vi "RT Read analogue FIFO queue data.vi"(9 "FIFO parameters":T2, 11 "RT Queues":T1) -> ()   [LabVIEW 2018]
doc: "This loop receives data from the FPGA via the FIFO\n\nThis loop performs no processing and just reads data from the FIFO and passes it onto the processing loop.\n\nThis is a mini state-machine with three states:\n* initialise - set parameters and reset variables to initial conditions\n* connect - check for FPGA FIFO connection\n* read data - read data on FIFO and stream to data processing loop\n\nInitial parameters are received when the loop is first called and therefore a RT machine reset is required to use different parameters"
uses:
  Type Defs/Analogue loop data.ctl
  Type Defs/FPGA reference.ctl
  Type Defs/Queues cluster.ctl
  ICL-LabVIEW_General/Message Scheduler/message scheduler.lvclass
  Analogue FIFO loop/Analogue FIFO loop states.ctl
  Queue VIs/De-queue RT FIFO loop element.vi
  Queue VIs/En-queue RT data element.vi
types:
  T1 = typedef "Queues cluster.ctl" = cluster{"RT Message":refnum<queue>, "RT Comms":refnum<queue>, "RT Data":refnum<queue>, "RT FIFO":refnum<queue>, "message scheduler":refnum<class "message scheduler.lvclass">}
  T2 = typedef "Analogue loop data.ctl" = cluster{"Params":cluster{"FPGA ref":T3, "Total Channels":u32}, "Variables":cluster{"FIFO wait counter":u16, "FIFO read trigger":u32}}
  T3 = typedef "FPGA reference.ctl" = refnum<k20>
  T4 = typedef "Analogue FIFO loop states.ctl" = enum16{"init", "message", "read", "stop"}
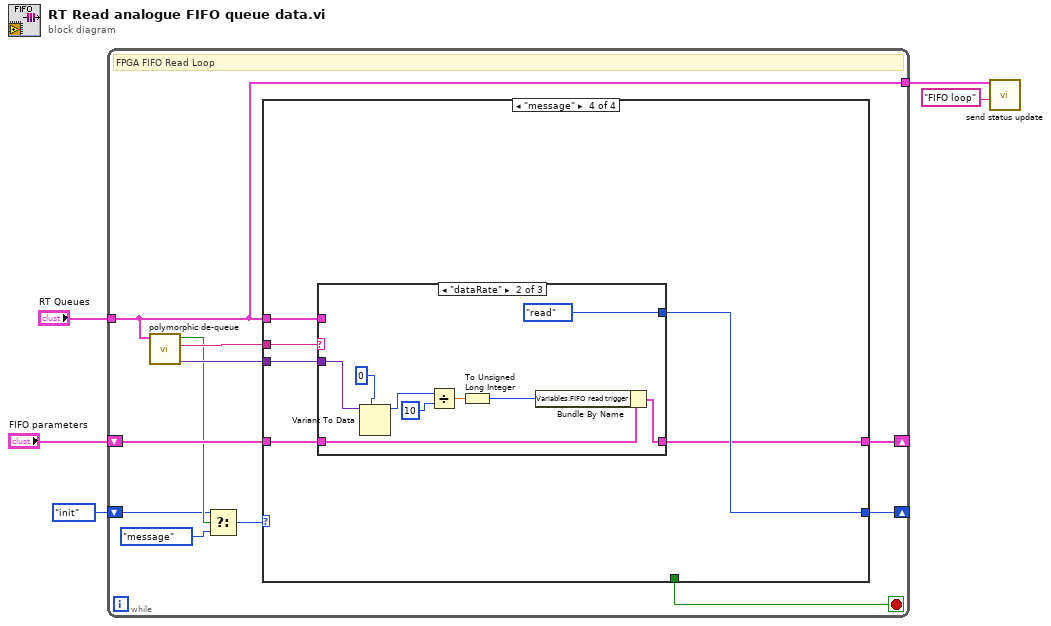
[diagram p0: block diagram]
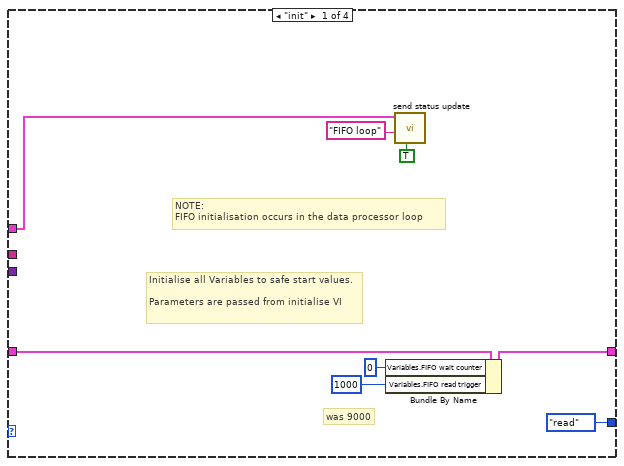
[diagram p2: hidden frame]
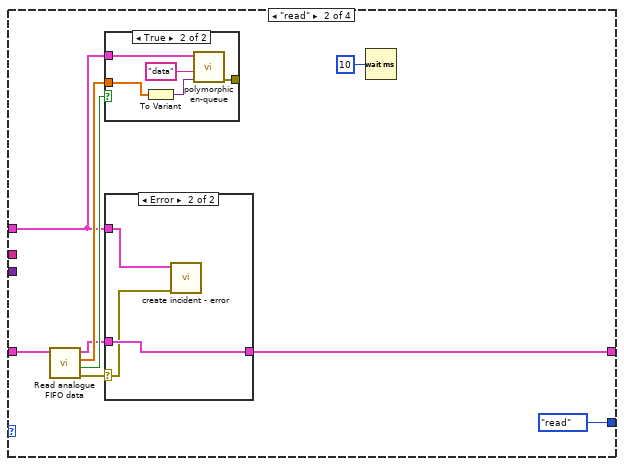
[diagram p3: hidden frame]
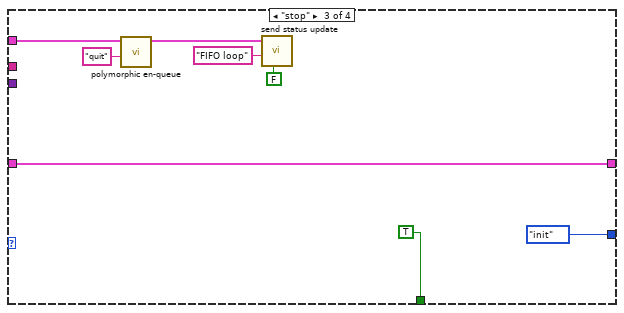
[diagram p6: hidden frame]
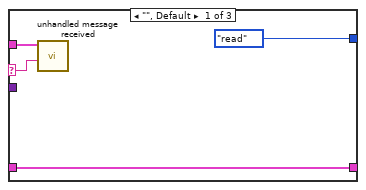
[diagram p7: hidden frame]
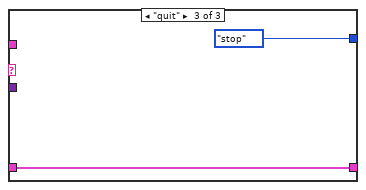
[diagram p8: hidden frame]
diagram:
  n1 = while {
    tunnel: "RT Queues" -> [w9]
    shift-right: [w16] -> _
    shift-left: Analogue_FIFO_loop_states."init" -> [w7]
    shift-right: [w15] -> _
    shift-left: "FIFO parameters" -> [w14]
    tunnel: [w9] -> w1
    stop <- w13 stop-if-true
    # "FPGA FIFO Read Loop"
    n2 = call-poly "polymorphic de-queue.vi"("RT Queues"=w9) -> ("Data"=w11:variant, "Message"=w10:string, "timed out?"=w8:bool)  [unwired: 7 in, 1 out]
    n3 = Select(t=w7, s=w8, f=Analogue_FIFO_loop_states."message") -> (s? t:f=w12:T4)
    n4 = case shown="\"message\"" w12 {
      tunnel: [Analogue_FIFO_loop_states."read" Analogue_FIFO_loop_states."read" Analogue_FIFO_loop_states."init" w56] -> w16
      tunnel: [w20 w29 w49 w51] -> w15
      tunnel: w14 -> [w19 w30 w49 w52]
      tunnel: w9 -> [w21 w28 w45 w53]
      tunnel: [_ _ TRUE _] -> w13
      tunnel: w11 -> [_ _ _ w55]
      tunnel: w10 -> [_ _ _ w54]
      frame "init" {
        # "was 9000"
        # "NOTE:\nFIFO initialisation occurs in the data processor loop"
        # "Initialise all Variables to safe start values.\n\nParameters are passed from initialise VI"
        n5 = Bundle By Name(cluster=w19, "Variables.FIFO wait counter"=u16 0, "Variables.FIFO read trigger"=u32 1000 ("y")) -> (w20:T2)
        n6 = call "send status update.vi"("status (F)"=TRUE, "subject"="FIFO loop" ("Message"), "RT Queues"=w21) -> ()  [unwired: 8 in, 1 out]
      }
      frame "read" {
        n7 = call "Read analogue FIFO data.vi"(11:w30) -> ("error out"=w31:errorcluster, "Data read"=w32:bool, "Data"=w33:sgl[], 3:w26:T2)  [unwired: 7 in]
        n8 = case shown="True" w32 {
          tunnel: w28 -> [_ w42]
          tunnel: w33 -> [_ w40]
          tunnel: [_ w38] -> _
          frame False {
          }
          frame True {
            n9 = To Variant(anything=w40) -> (Variant=w39:variant)
            n10 = call-poly "polymorphic en-queue.vi"("Data"=w39, "Message"="data", "RT Queues"=w42) -> ("error out"=w38:errorcluster)  [unwired: 6 in, 2 out]
          }
        }
        n11 = case shown="Error" w31 {
          selector: w31 -> [_ w36]
          tunnel: [w34 w37] -> w29
          tunnel: w26 -> [w34 w37]
          tunnel: w28 -> [_ w35]
          frame No Error {
          }
          frame Error {
            n12 = call "create incident - error.vi"("error"=w36, "RT Queues"=w35) -> ()  [unwired: 9 in, 1 out]
          }
        }
        n13 = Wait (ms)(milliseconds to wait=u32 10) -> ()  [unwired: 1 out]
      }
      frame "stop" {
        n14 = call-poly "polymorphic en-queue.vi"("Message"="quit", "RT Queues"=w45) -> ("RT Queues out"=w44:T1)  [unwired: 7 in, 2 out]
        n15 = call "send status update.vi"("status (F)"=FALSE, "subject"="FIFO loop" ("Message"), "RT Queues"=w44) -> ()  [unwired: 8 in, 1 out]
      }
      frame "message" {
        n16 = case shown="\"dataRate\"" w54 {
          selector: w54 -> [w58 _ _]
          tunnel: w55 -> [_ w67 _]
          tunnel: [Analogue_FIFO_loop_states."read" Analogue_FIFO_loop_states."read" Analogue_FIFO_loop_states."stop"] -> w56
          tunnel: w53 -> [w59 _ _]
          tunnel: [w57 w68 w70] -> w51
          tunnel: w52 -> [w57 w69 w70]
          frame "", Default {
            n17 = call "unhandled message received.vi"("unhandled message"=w58, "RT Queues"=w59) -> ()  [unwired: 10 in]
          }
          frame "dataRate" {
            n18 = Variant To Data(type=u16 0 ("Variables.FIFO read trigger"), Variant=w67) -> (data=w64:u16)  [unwired: 1 in, 1 out]
            n19 = Divide(x=w64, y=u16 10) -> (x/y=w62:dbl)
            n20 = To Unsigned Long Integer(number=w62) -> (unsigned 32bit integer=w61:u32)
            n21 = Bundle By Name(cluster=w69, "Variables.FIFO read trigger"=w61) -> (w68:T2)
          }
          frame "quit" {
          }
        }
      }
    }
  }
  n22 = call "send status update.vi"("subject"="FIFO loop" ("Message"), "RT Queues"=w1) -> ()  [unwired: 9 in, 1 out]
